vi "NI_9222_Anologue_DAQ_FPGA_Host.vi"() -> ()   [LabVIEW 2013]
uses:
  <vilib>/rvi/interface/nirviOpenFPGA/nirviOpenFPGA.xnode
  <vilib>/rvi/interface/nirviReadWriteControl/nirviReadWriteControl.xnode
  <vilib>/rvi/interface/Simulation/niFpgaSimulationCallBeginRW.vi
  <vilib>/rvi/errors/niLvFpgaAdjustHostInterfaceError.vi
  <vilib>/rvi/interface/nirviMethod/nirviMethod.xnode
  <vilib>/rvi/errors/niLvFpgaMergeErrorWithErrorCode.vi
  <vilib>/rvi/interface/nirviCloseFPGA/nirviCloseFPGA.xnode
  <vilib>/rvi/interface/nirviMethod/StockFPGA_InlinedMethodWaitForSingleIRQ.vi
  <vilib>/FPGAPlugInAG/Dynamic/niLvFpga_WaitOnIrq_Dynamic.vi
  <vilib>/FPGAPlugInAG/Dynamic/niLvFpga_AcknowledgeIrq_Dynamic.vi
  NI_9222_Anologue_DAQ_FPGA.vi
  <vilib>/FPGAPlugInAG/Dynamic/niLvFpga_StartFifo_Dynamic.vi
  <vilib>/FPGAPlugInAG/Dynamic/niLvFpga_Close_Dynamic.vi
  <vilib>/FPGAPlugInAG/Dynamic/niLvFpga_ReadFifo_Dynamic.vi
  <vilib>/userDefined/High Color/nirio_resource_hc.ctl
panel:
  out "appended array":fxp<+/-,24,5>[][](array[numeric])
  out "FPGA Error Out":errorcluster
  in  "RIO Device":T1="RIO0"
  out "Timed Out":bool
  out "Sample Gated":bool
  out "Overwrite":bool
  in  "stop":bool
  in  "Sample Period (uSec)":u32=2
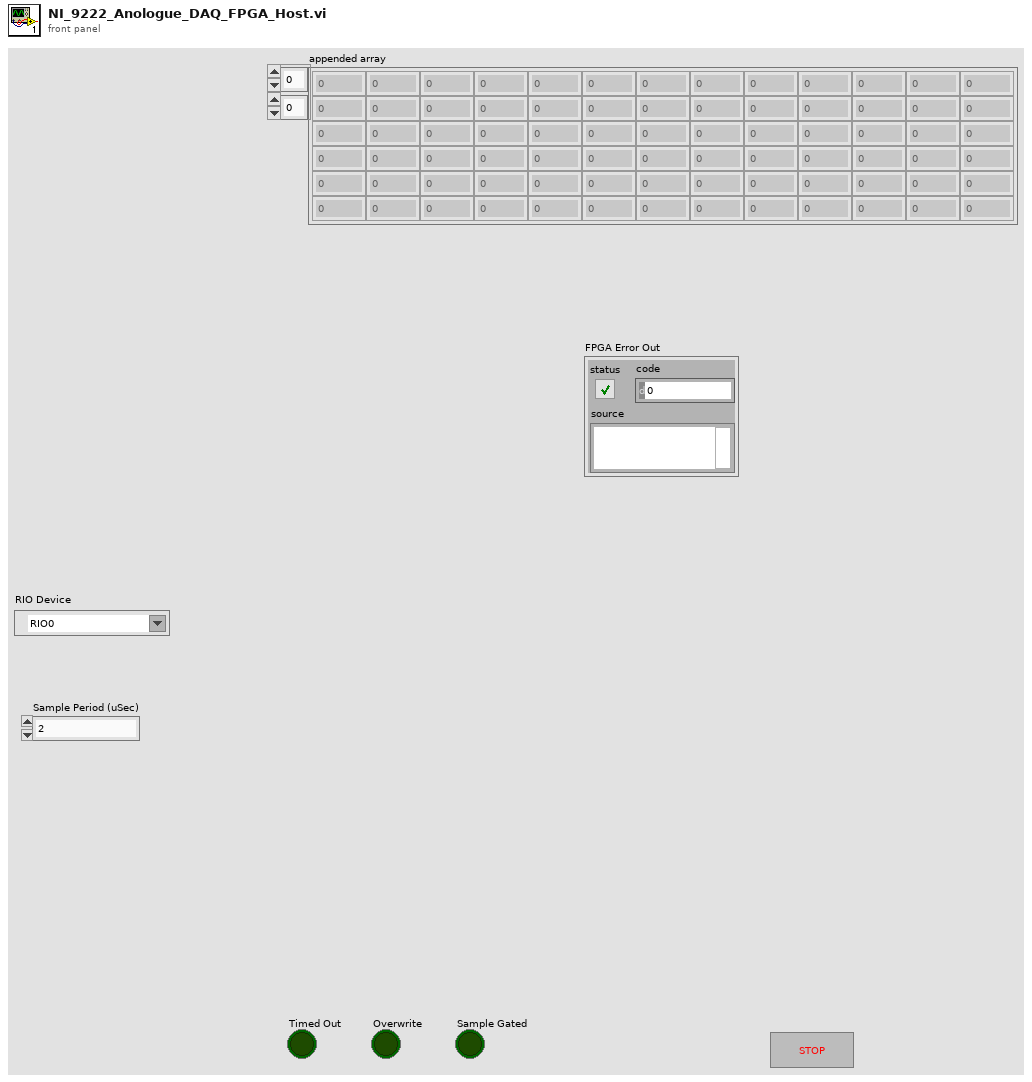
[diagram p1: front panel]
types:
  T1 = typedef "nirio_resource_hc.ctl" = tag
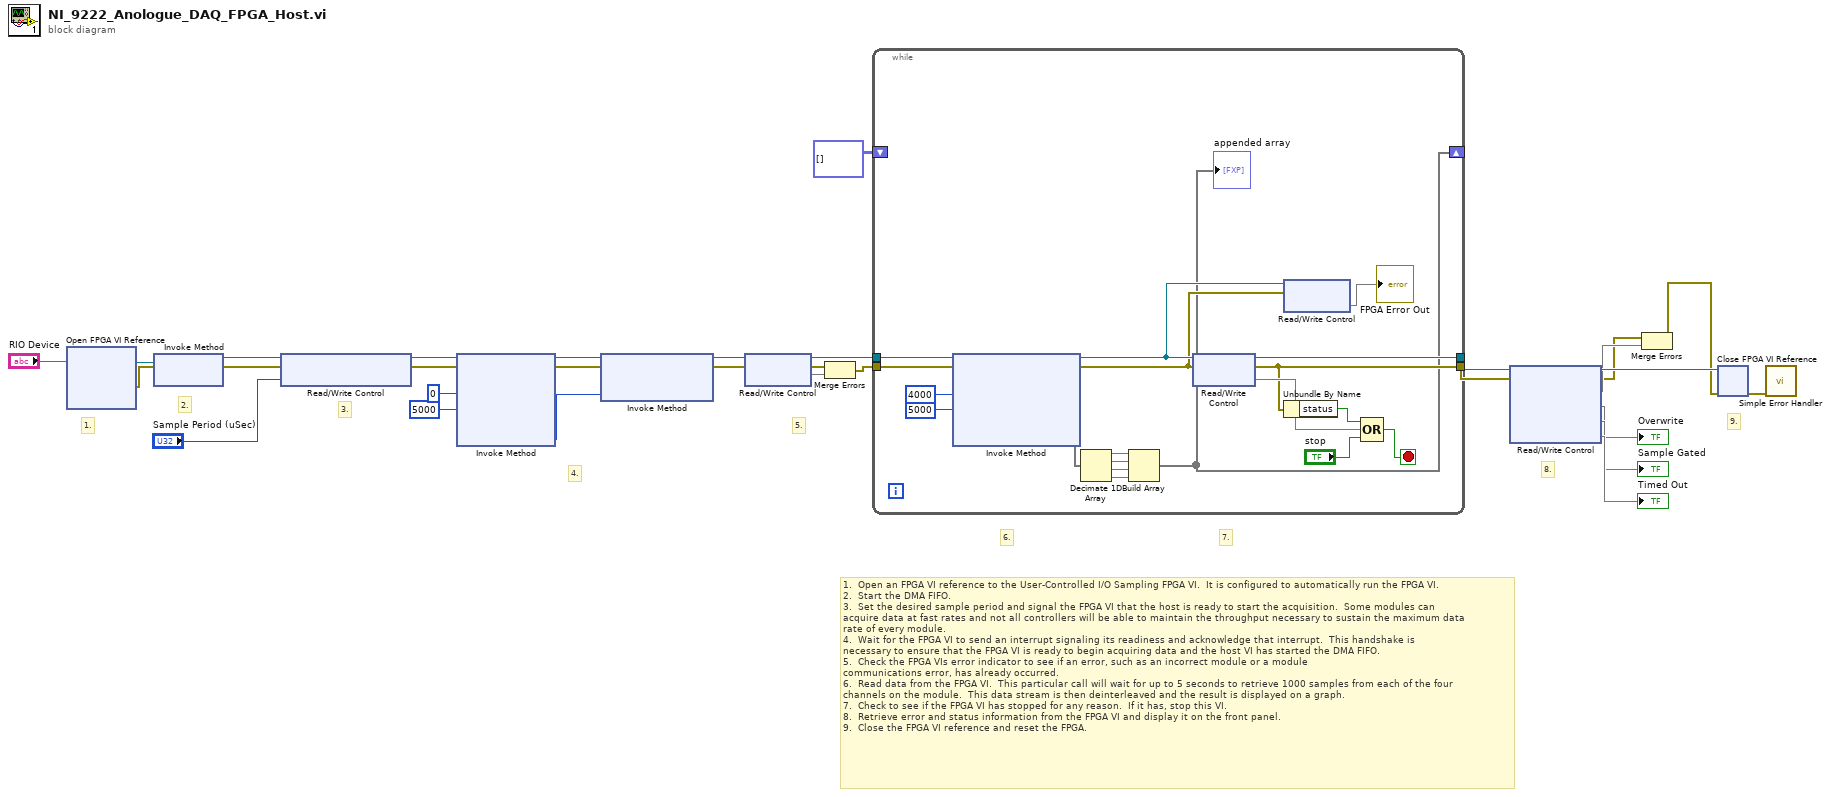
[diagram p0: block diagram]
diagram:
  # "7."
  # "6."
  # "5."
  # "4."
  # "1.  Open an FPGA VI reference to the User-Controlled I/O Sampling FPGA VI.  It is configured to automatically run the FPGA VI.\n2.  Start the DMA FIFO.\n3.  Set the desired sample period and signal the FPGA VI that the host is ready to start the acquisition.  Some modules can \nacquire data at fast rates and not all controllers will be able to maintain the throughput necessary to sustain the maximum data \nrate of every module.\n4.  Wait for the FPGA VI to send an interrupt signaling its readiness and acknowledge that interrupt.  This handshake is \nnecessary to ensure that the FPGA VI is ready to begin acquiring data and the host VI has started the DMA FIFO.\n5.  Check the FPGA VIs error indicator to see if an error, such as an incorrect module or a module \ncommunications error, has already occurred.\n6.  Read data from the FPGA VI.  This particular call will wait for up to 5 seconds to retrieve 1000 samples from each of the four \nchannels on the module.  This data stream is then deinterleaved and the result is displayed on a graph.\n7.  Check to see if the FPGA VI has stopped for any reason.  If it has, stop this VI.\n8.  Retrieve error and status information from the FPGA VI and display it on the front panel.\n9.  Close the FPGA VI reference and reset the FPGA."
  # "9."
  # "8."
  # "3."
  # "2."
  # "1."
  n1 = xnode "Open FPGA VI Reference"("resource name"="RIO Device") -> ("FPGA VI Reference Out"=w28:refnum<k20>, "error out"=w29:errorcluster)  [unwired: 1 in]
  n2 = xnode "Invoke Method"("FPGA VI Reference In"=w28, "error in"=w29) -> ("FPGA VI Reference Out"=w27:refnum<k20>, "error out"=w26:errorcluster)
  n3 = xnode "Read/Write Control"("FPGA VI Reference In"=w27, "error in"=w26, "Sample Period (uSec)"="Sample Period (uSec)") -> ("FPGA VI Reference Out"=w11:refnum<k20>, "error out"=w10:errorcluster)
  n4 = xnode "Invoke Method"("FPGA VI Reference In"=w11, "error in"=w10, "IRQ Number(s)"=0, "Timeout (ms)"=5000) -> ("FPGA VI Reference Out"=w8:refnum<k20>, "error out"=w9:errorcluster, "IRQ(s) Asserted"=w5:i32)  [unwired: 1 out]
  n5 = xnode "Invoke Method"("FPGA VI Reference In"=w8, "error in"=w9, "IRQ Number(s)"=w5) -> ("FPGA VI Reference Out"=w7:refnum<k20>, "error out"=w6:errorcluster)
  n6 = xnode "Read/Write Control"("FPGA VI Reference In"=w7, "error in"=w6) -> ("FPGA VI Reference Out"=w12:refnum<k20>, "error out"=w14:errorcluster, "Error Out"=w13)
  n7 = Merge Errors(w14, w13) -> (w15:errorcluster)
  n8 = while {
    tunnel: w12 -> [w38]
    tunnel: w15 -> [w49]
    tunnel: [w39] -> w25
    tunnel: [w36] -> w24
    shift-right: [w31] -> _
    shift-left: fxp<+/-,24,5>[][] [] -> [_]
    stop <- w37 stop-if-true
    n9 = xnode "Invoke Method"("FPGA VI Reference In"=w38, "error in"=w49, "Number of Elements"=u32 4000, "Timeout (ms)"=5000) -> ("FPGA VI Reference Out"=w34:refnum<k20>, "error out"=w33:errorcluster, "Data"=w46:void[])  [unwired: 1 out]
    n10 = Decimate 1D Array(w46) -> (w35:void[], w43:void[], w44:void[], w45:void[])
    n11 = Build Array(w35, w43, w44, w45) -> (w31:void[])
    "appended array" <- w31
    n12 = xnode "Read/Write Control"("FPGA VI Reference In"=w34, "error in"=w33) -> ("FPGA VI Reference Out"=w39:refnum<k20>, "error out"=w36:errorcluster, "Stopped"=w41)
    n13 = xnode "Read/Write Control"("FPGA VI Reference In"=w34, "error in"=w33) -> ("Error Out"=→"FPGA Error Out")  [unwired: 2 out]
    n14 = Unbundle By Name(w36) -> ("status"=w40:bool)
    n15 = Compound Arithmetic op=OR(w40, w41, "stop") -> (w37:bool)
  }
  n16 = xnode "Read/Write Control"("FPGA VI Reference In"=w25, "error in"=w24) -> ("FPGA VI Reference Out"=w23:refnum<k20>, "error out"=w17:errorcluster, "Error Out"=w18, "Overwrite"=→"Overwrite", "Sample Gated"=→"Sample Gated", "Timed Out"=→"Timed Out")
  n17 = Merge Errors(w17, w18) -> (w2:errorcluster)
  n18 = xnode "Close FPGA VI Reference"("FPGA VI Reference In"=w23, "error in"=w2) -> ("error out"=w16:errorcluster)
  n19 = call <vilib>:"Simple Error Handler.vi"("error in (no error)"=w16) -> ()  [unwired: 4 in, 5 out]
